vi "Remove JSONtext from palette.vi"() -> ()   [LabVIEW 2017]
uses:
  <vilib>/Palette API/Palette Menu/Public Type Define/Palette Data.ctl
  <vilib>/Palette API/Palette Menu/Public Type Define/View Format.ctl
  <vilib>/Palette API/Palette Menu/Public Type Define/Items.ctl
  <vilib>/Palette API/Palette Menu/Public Type Define/Item.ctl
  <vilib>/Palette API/Palette Menu/Public Type Define/Help Info.ctl
  <vilib>/Palette API/Palette Menu/Public Type Define/Synchronize Info.ctl
  <vilib>/Palette API/Palette Menu/Public Type Define/Palette type.ctl
  <vilib>/Palette API/Palette Menu/Palette Menu.lvlib
panel:
  out "palette data":T1={"display name"="", "view format"=0, "palette width"=4, "items"=[], "256 color icon"=bytes[0], "B&W color icon"=bytes[0], "help information"={"help tag"="", "help file path "=path ""}, "palette description"="", "synchronize information"={"synchronize with directory"=FALSE, "synchronize directory path"=path ""}} {"view format" items=["Icons", "Text", "Icons and Text"]}
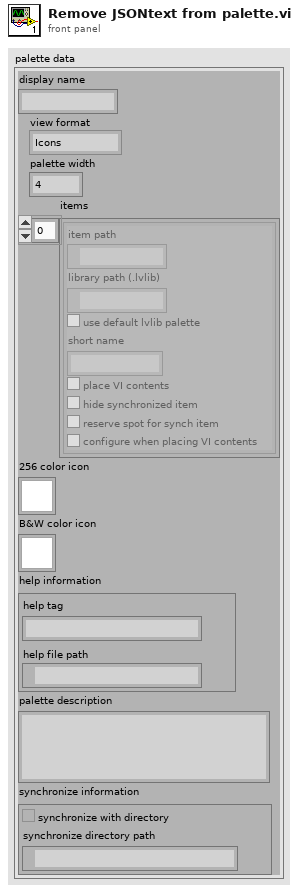
[diagram p1: front panel]
types:
  T1 = typedef "Palette Menu.lvlib/Palette Data.ctl" = cluster{"display name":string, "view format":T2, "palette width":i16, "items":T3, "256 color icon":picture, "B&W color icon":picture, "help information":T5, "palette description":string, "synchronize information":T6}
  T2 = typedef "Palette Menu.lvlib/View Format.ctl" = u16
  T3 = typedef "Palette Menu.lvlib/Items.ctl" = T4[]
  T4 = typedef "Palette Menu.lvlib/Item.ctl" = cluster{"item path":path, "library path (.lvlib)":path, "use default lvlib palette":bool, "short name":string, "place VI contents":bool, "hide synchronized item":bool, "reserve spot for synch item":bool, "configure when placing VI contents":bool}
  T5 = typedef "Palette Menu.lvlib/Help Info.ctl" = cluster{"help tag":string, "help file path ":path}
  T6 = typedef "Palette Menu.lvlib/Synchronize Info.ctl" = cluster{"synchronize with directory":bool, "synchronize directory path":path}
  T7 = typedef "Palette Menu.lvlib/Palette type.ctl" = i32
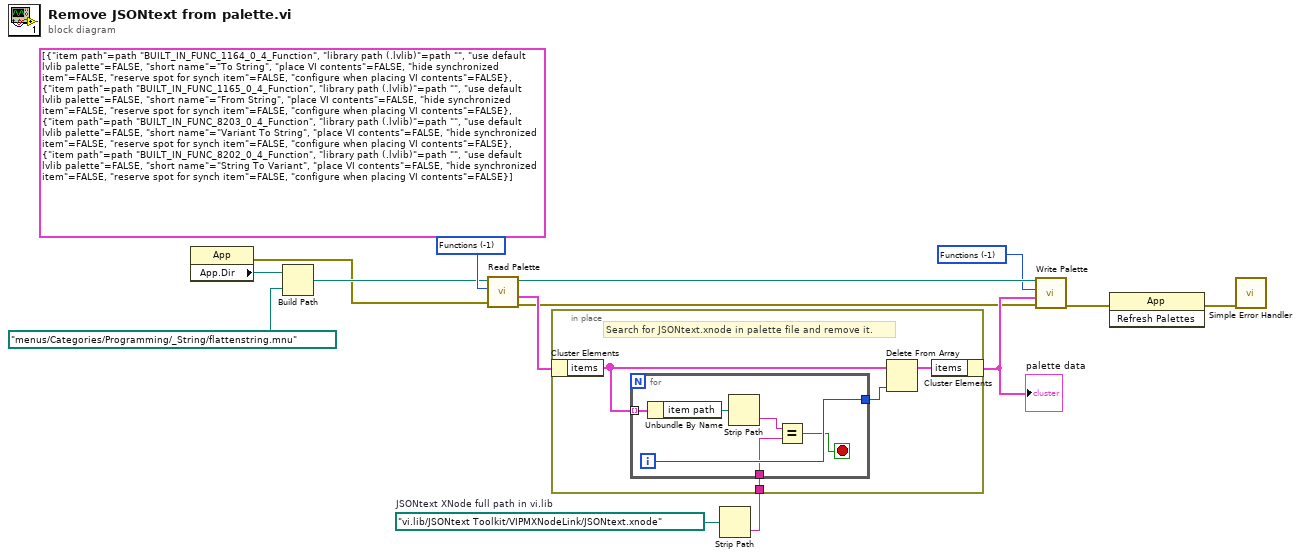
[diagram p0: block diagram]
diagram:
  (unwired) T4[] [{"item path"=path "BUILT_IN_FUNC_1164_0_4_Function", "library path (.lvlib)"=path "", "use default lvlib palette"=FALSE, "short name"="To String", "place VI contents"=FALSE, "hide synchronized item"=FALSE, "reserve spot for synch item"=FALSE, "configure when placing VI contents"=FALSE}, {"item path"=path "BUILT_IN_FUNC_1165_0_4_Function", "library path (.lvlib)"=path "", "use default lvlib palette"=FALSE, "short name"="From String", "place VI contents"=FALSE, "hide synchronized item"=FALSE, "reserve spot for synch item"=FALSE, "configure when placing VI contents"=FALSE}, {"item path"=path "BUILT_IN_FUNC_8203_0_4_Function", "library path (.lvlib)"=path "", "use default lvlib palette"=FALSE, "short name"="Variant To String", "place VI contents"=FALSE, "hide synchronized item"=FALSE, "reserve spot for synch item"=FALSE, "configure when placing VI contents"=FALSE}, {"item path"=path "BUILT_IN_FUNC_8202_0_4_Function", "library path (.lvlib)"=path "", "use default lvlib palette"=FALSE, "short name"="String To Variant", "place VI contents"=FALSE, "hide synchronized item"=FALSE, "reserve spot for synch item"=FALSE, "configure when placing VI contents"=FALSE}] ("items")
  w3 = T7 -1 items=["Functions"=-1, "Controls"=-2] ("palette type")
  w9 = path "vi.lib/JSONtext Toolkit/VIPMXNodeLink/JSONtext.xnode"  # JSONtext XNode full path in vi.lib
  w14 = T7 -1 items=["Functions"=-1, "Controls"=-2] ("palette type")
  n1 = property class="App"() -> (error out=w2:errorcluster, "App.Dir"=w11:path)  [unwired: 2 in, 1 out]
  n2 = Build Path(base path=w11, name or relative path=path "menus/Categories/Programming/_String/flattenstring.mnu") -> (appended path=w12:path)
  n3 = call <vilib>:"Read Palette.vi"("error in (no error)"=w2, "palette type"=w14, "palette path"=w12) -> ("error out"=w1:errorcluster, "palette data"=w10:T1, "duplicate palette path"=w7:path)  [unwired: 1 in, 5 out]
  n4 = Strip Path(path=w9) -> (name=w6:string)  [unwired: 1 out]
  n5 = in-place {
    in-place-border: w6 -> [w15]
    # "Search for JSONtext.xnode in palette file and remove it."
    n6 = in-place-cluster #1(w10) -> ("items"=w17:T3)
    n7 = for {
      tunnel: w17 -> [w24] mode=indexing
      tunnel: [w22] -> w18
      tunnel: w15 -> [w20]
      i -> [w22]
      stop <- w19 stop-if-true
      n8 = Unbundle By Name(w24) -> ("item path"=w23:path)
      n9 = Strip Path(path=w23) -> (name=w21:string)  [unwired: 1 out]
      n10 = Equal?(x=w21, y=w20) -> (x = y?=w19:bool)
    }
    n11 = Delete From Array(array=w17, index=w18) -> (array with subset deleted=w16:T3)  [unwired: 1 in, 1 out]
    n12 = in-place-cluster #1("items"=w16) -> (w8:T1)
  }
  "palette data" <- w8
  n13 = call <vilib>:"Write Palette.vi"("error in (no error)"=w1, "palette data"=w8, "palette type"=w3, "palette path"=w7) -> ("error out"=w4:errorcluster)  [unwired: 1 in, 6 out]
  n14 = invoke class="App" method="Refresh Palettes"(error in=w4) -> (error out=w5:errorcluster)  [unwired: 2 in, 2 out]
  n15 = call <vilib>:"Simple Error Handler.vi"("error in (no error)"=w5) -> ()  [unwired: 1 in, 8 out]
